vi "Get Time Strings.vi"() -> (0 "File YMD":string, 1 "File YMD HMS":string, 2 "YMD HMS":string, 3 "YMD HMS with milliseconds":string)   [LabVIEW 2026, in "Time Utils.lvlib"]
uses:
  Time Utils.lvlib
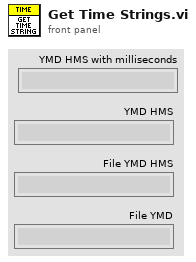
[diagram p1: front panel]
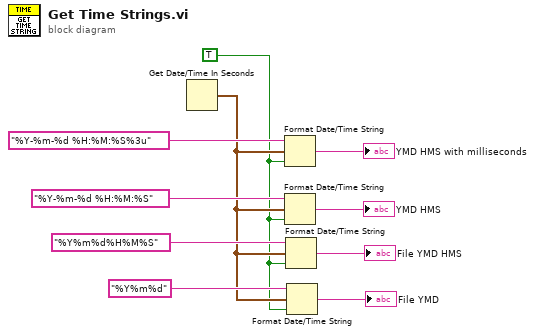
[diagram p0: block diagram]
diagram:
  w1 = TRUE ("UTC format")
  n1 = Get Date/Time In Seconds() -> (seconds since 1Jan1904=w2:timestamp)
  n2 = Format Date/Time String(time format string (%c)="%Y-%m-%d %H:%M:%S%3u", seconds (now)=w2, UTC format=w1) -> (date/time string=→"YMD HMS with milliseconds":string)
  n3 = Format Date/Time String(time format string (%c)="%Y-%m-%d %H:%M:%S", seconds (now)=w2, UTC format=w1) -> (date/time string=→"YMD HMS":string)
  n4 = Format Date/Time String(time format string (%c)="%Y%m%d%H%M%S", seconds (now)=w2, UTC format=w1) -> (date/time string=→"File YMD HMS":string)
  n5 = Format Date/Time String(time format string (%c)="%Y%m%d", seconds (now)=w2, UTC format=w1) -> (date/time string=→"File YMD":string)
